vi "Check Image Deplication.vi"(8 "error in (no error)":errorcluster, 10 "IndexOfImages":i32, 11 "FileOperation in":refnum<class "FileOperation.lvclass">) -> (0 "error out":errorcluster, 2 "Effective?(True)":bool, 3 "FileOperation out":refnum<class "FileOperation.lvclass">)   [LabVIEW 2015, in "FileOperation.lvclass"]
uses:
  FileOperation.lvclass
  FileOperation.lvclass/FileOperation.ctl
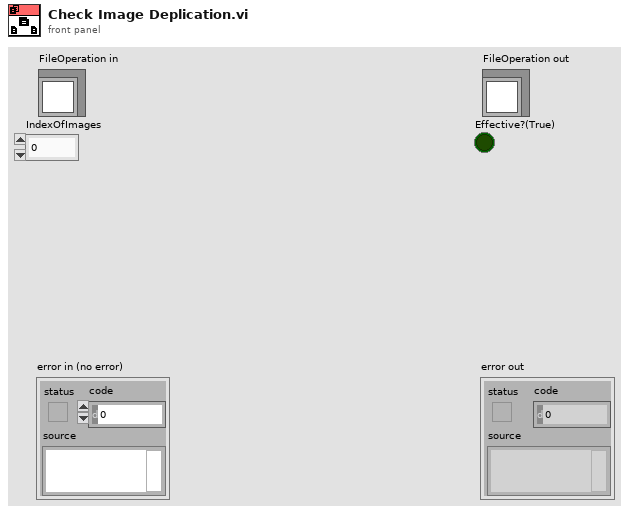
[diagram p1: front panel]
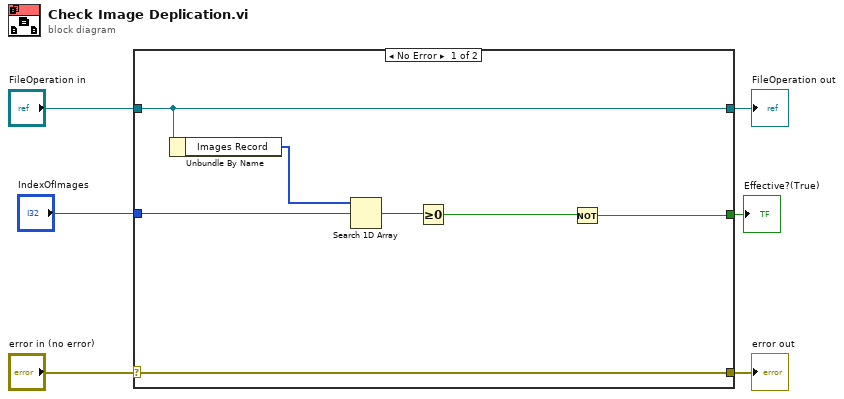
[diagram p0: block diagram]
diagram:
  n1 = case shown="No Error" "error in (no error)" {
    selector: "error in (no error)" -> [w9 w15]
    tunnel: [w9 w15] -> w5
    tunnel: [w13 w14] -> w3
    tunnel: "FileOperation in" -> [w13 w14]
    tunnel: "IndexOfImages" -> [w11 _]
    tunnel: [w7 _] -> w1
    frame No Error {
      n2 = Unbundle By Name(w13) -> ("Images Record"=w12:i32[])
      n3 = Search 1D Array(1D array=w12, element=w11) -> (index of element=w10:i32)  [unwired: 1 in]
      n4 = Greater Or Equal To 0?(x=w10) -> (x >= 0?=w8:bool)
      n5 = Not(x=w8) -> (.not. x?=w7:bool)
    }
    frame Error {
    }
  }
  "error out" <- w5
  "FileOperation out" <- w3
  "Effective?(True)" <- w1
